vi "GUI_Magspec_BELLA_waterfall.vi"() -> ()   [LabVIEW 2013]
uses:
  shared programs/GUI_Template/GUI_master/tcp_new_data_event.ctl
  shared programs/GUI_Template/GUI_master/tcp new data cluster.ctl
  General/Device GUIs/GUI_Cameras/color tables/image color table presets.ctl
  shared programs/MySQL/Preset Query Enum.ctl
  <vilib>/Analysis/2dsp.llb/Decimate (single shot, DBL).vi
  <vilib>/Utility/tcp.llb/UDP Multicast Read-Only Open.vi
  <vilib>/vision/NI_Vision_Development_Module.lvlib
  <vilib>/Analysis/NI_AALPro.lvlib
panel:
  in  "Color table":T1=enum."BYR enhance low"
  out "Momentum 3":dbl=8.582505 caption="Momentum (GeV/c)" min=0.0 max=0.0 format="%#.1f"
  out "Momentum 4":dbl=7.19823 caption="Momentum (GeV/c)" min=0.0 max=0.0 format="%#.1f"
  out "Momentum 5":dbl=5.675527499999999 caption="Momentum (GeV/c)" min=0.0 max=0.0 format="%#.1f"
  out "Momentum 6":dbl=4.36046625 caption="Momentum (GeV/c)" min=0.0 max=0.0 format="%#.1f"
  out "C":T2(plugin-control) caption="C cam"
  out "D":T2(plugin-control) caption="D Cam"
  out "E":T2(plugin-control) caption="E Cam"
  out "Momentum 7":dbl=4.014397499999999 caption="Momentum (GeV/c)" min=0.0 max=0.0 format="%#.1f"
  out "Momentum 8":dbl=2.97619125 caption="Momentum (GeV/c)" min=0.0 max=0.0 format="%#.1f"
  out "Momentum 9":dbl=2.0210415 caption="Momentum (GeV/c)" min=0.0 max=0.0 format="%#.1f"
  out "Momentum 10":dbl=1.218162 caption="Momentum (GeV/c)" min=0.0 max=0.0 format="%#.1f"
  out "Momentum 11":dbl=0.67829475 caption="Momentum (GeV/c)" min=0.0 max=0.0 format="%#.1f"
  out "Momentum 12":dbl=0.276855 caption="Momentum (GeV/c)" min=0.0 max=0.0 format="%#.1f"
  out "Momentum 13":dbl=0.06921375 caption="Momentum (GeV/c)" min=0.0 max=0.0 format="%#.1f"
  out "Momentum 14":dbl=0.0055371 caption="Momentum (GeV/c)" min=0.0 max=0.0 format="%#.1f"
  out "F":T2(plugin-control) caption="F Cam"
  out "G":T2(plugin-control) caption="G Cam"
  out "H":T2(plugin-control) caption="H Cam"
  out "I":T2(plugin-control) caption="I Cam"
  out "J":T2(plugin-control) caption="J Cam"
  out "K":T2(plugin-control) caption="K Cam"
  out "L":T2(plugin-control) caption="L Cam"
  out "Momentum 2":dbl=9.5514975 caption="Momentum (GeV/c)" min=0.0 max=0.0 format="%#.1f"
  out "B":T2(plugin-control) caption="B Cam"
  out "Momentum 1":dbl=26.301225 caption="Momentum (GeV/c)" min=0.0 max=0.0 format="%#.1f"
  out "EBeam":T2(plugin-control) caption="Beam Profile"
  out "A":T2(plugin-control) caption="A Cam"
  in  "Max P [MeV/c]":dbl=6000.0
  out "ROI interpolated":cluster{"yi":dbl[], dbl[]}(graph)
  out "rough calcs out":T3={"peak charge (a.u.)"=nan, "momentum at peak (MeV/c)"=nan, "FWHM (MeV/c)"=nan, "Background"=nan, "sum"=0.0}
  in  "proper stitch":bool=TRUE
  out "Intensity Graph 6":dbl[][](graph)
  in  "Field::14":dbl=2.76855 caption="B Field (mT)" min=0.0 max=0.0 format="%_4f"
  out "Boolean":bool
  in  "options":T4={"B field [mT]"=400.0, "Max P [MeV/c]"=400.0, "filter rank"=1}
  out "ShotNumber":i32
  out "data":string[][](array[string])
  in  "rank for LPF":i32=2
  out "Waveform Graph":dbl[](graph)
  in  "HorizontalLineout::12":dbl[](array[numeric]) caption="HorizontalLineout MagSpecA"
  in  "HorizontalLineout::11":dbl[](array[numeric]) caption="HorizontalLineout MagSpecA"
  in  "HorizontalLineout::10":dbl[](array[numeric]) caption="HorizontalLineout MagSpecA"
  in  "HorizontalLineout::9":dbl[](array[numeric]) caption="HorizontalLineout MagSpecA"
  in  "HorizontalLineout::8":dbl[](array[numeric]) caption="HorizontalLineout MagSpecA"
  in  "HorizontalLineout::7":dbl[](array[numeric]) caption="HorizontalLineout MagSpecA"
  in  "HorizontalLineout::6":dbl[](array[numeric]) caption="HorizontalLineout MagSpecA"
  in  "HorizontalLineout::5":dbl[](array[numeric]) caption="HorizontalLineout MagSpecA"
  in  "HorizontalLineout::4":dbl[](array[numeric]) caption="HorizontalLineout MagSpecA"
  in  "HorizontalLineout::3":dbl[](array[numeric]) caption="HorizontalLineout MagSpecA"
  in  "HorizontalLineout::2":dbl[](array[numeric]) caption="HorizontalLineout MagSpecA"
  in  "HorizontalLineout::1":dbl[](array[numeric]) caption="HorizontalLineout MagSpecA"
  in  "GUIdevice 12":string="MagSpecL"
  in  "GUIdevice 11":string="MagSpecK"
  in  "GUIdevice 10":string="MagSpecJ"
  in  "GUIdevice 9":string="MagSpecI"
  in  "GUIdevice 8":string="MagSpecH"
  in  "GUIdevice 7":string="MagSpecG"
  in  "GUIdevice 6":string="MagSpecF"
  in  "GUIdevice 5":string="MagSpecE"
  in  "GUIdevice 4":string="MagSpecD"
  in  "GUIdevice 3":string="MagSpecC"
  in  "GUIdevice 2":string="MagSpecB"
  in  "GUIdevice 1":string="MagSpecA"
  in  "GUIdevice 14":string="BELLA_HallProbe"
  out "error IO 2":errorcluster
  out "tcp data event":T5
  in  "stop":bool
  # "AA side"
  # "B\nT\nM"
  # "T\no\np"
  # "Parking side"
  # "Beam Axis"
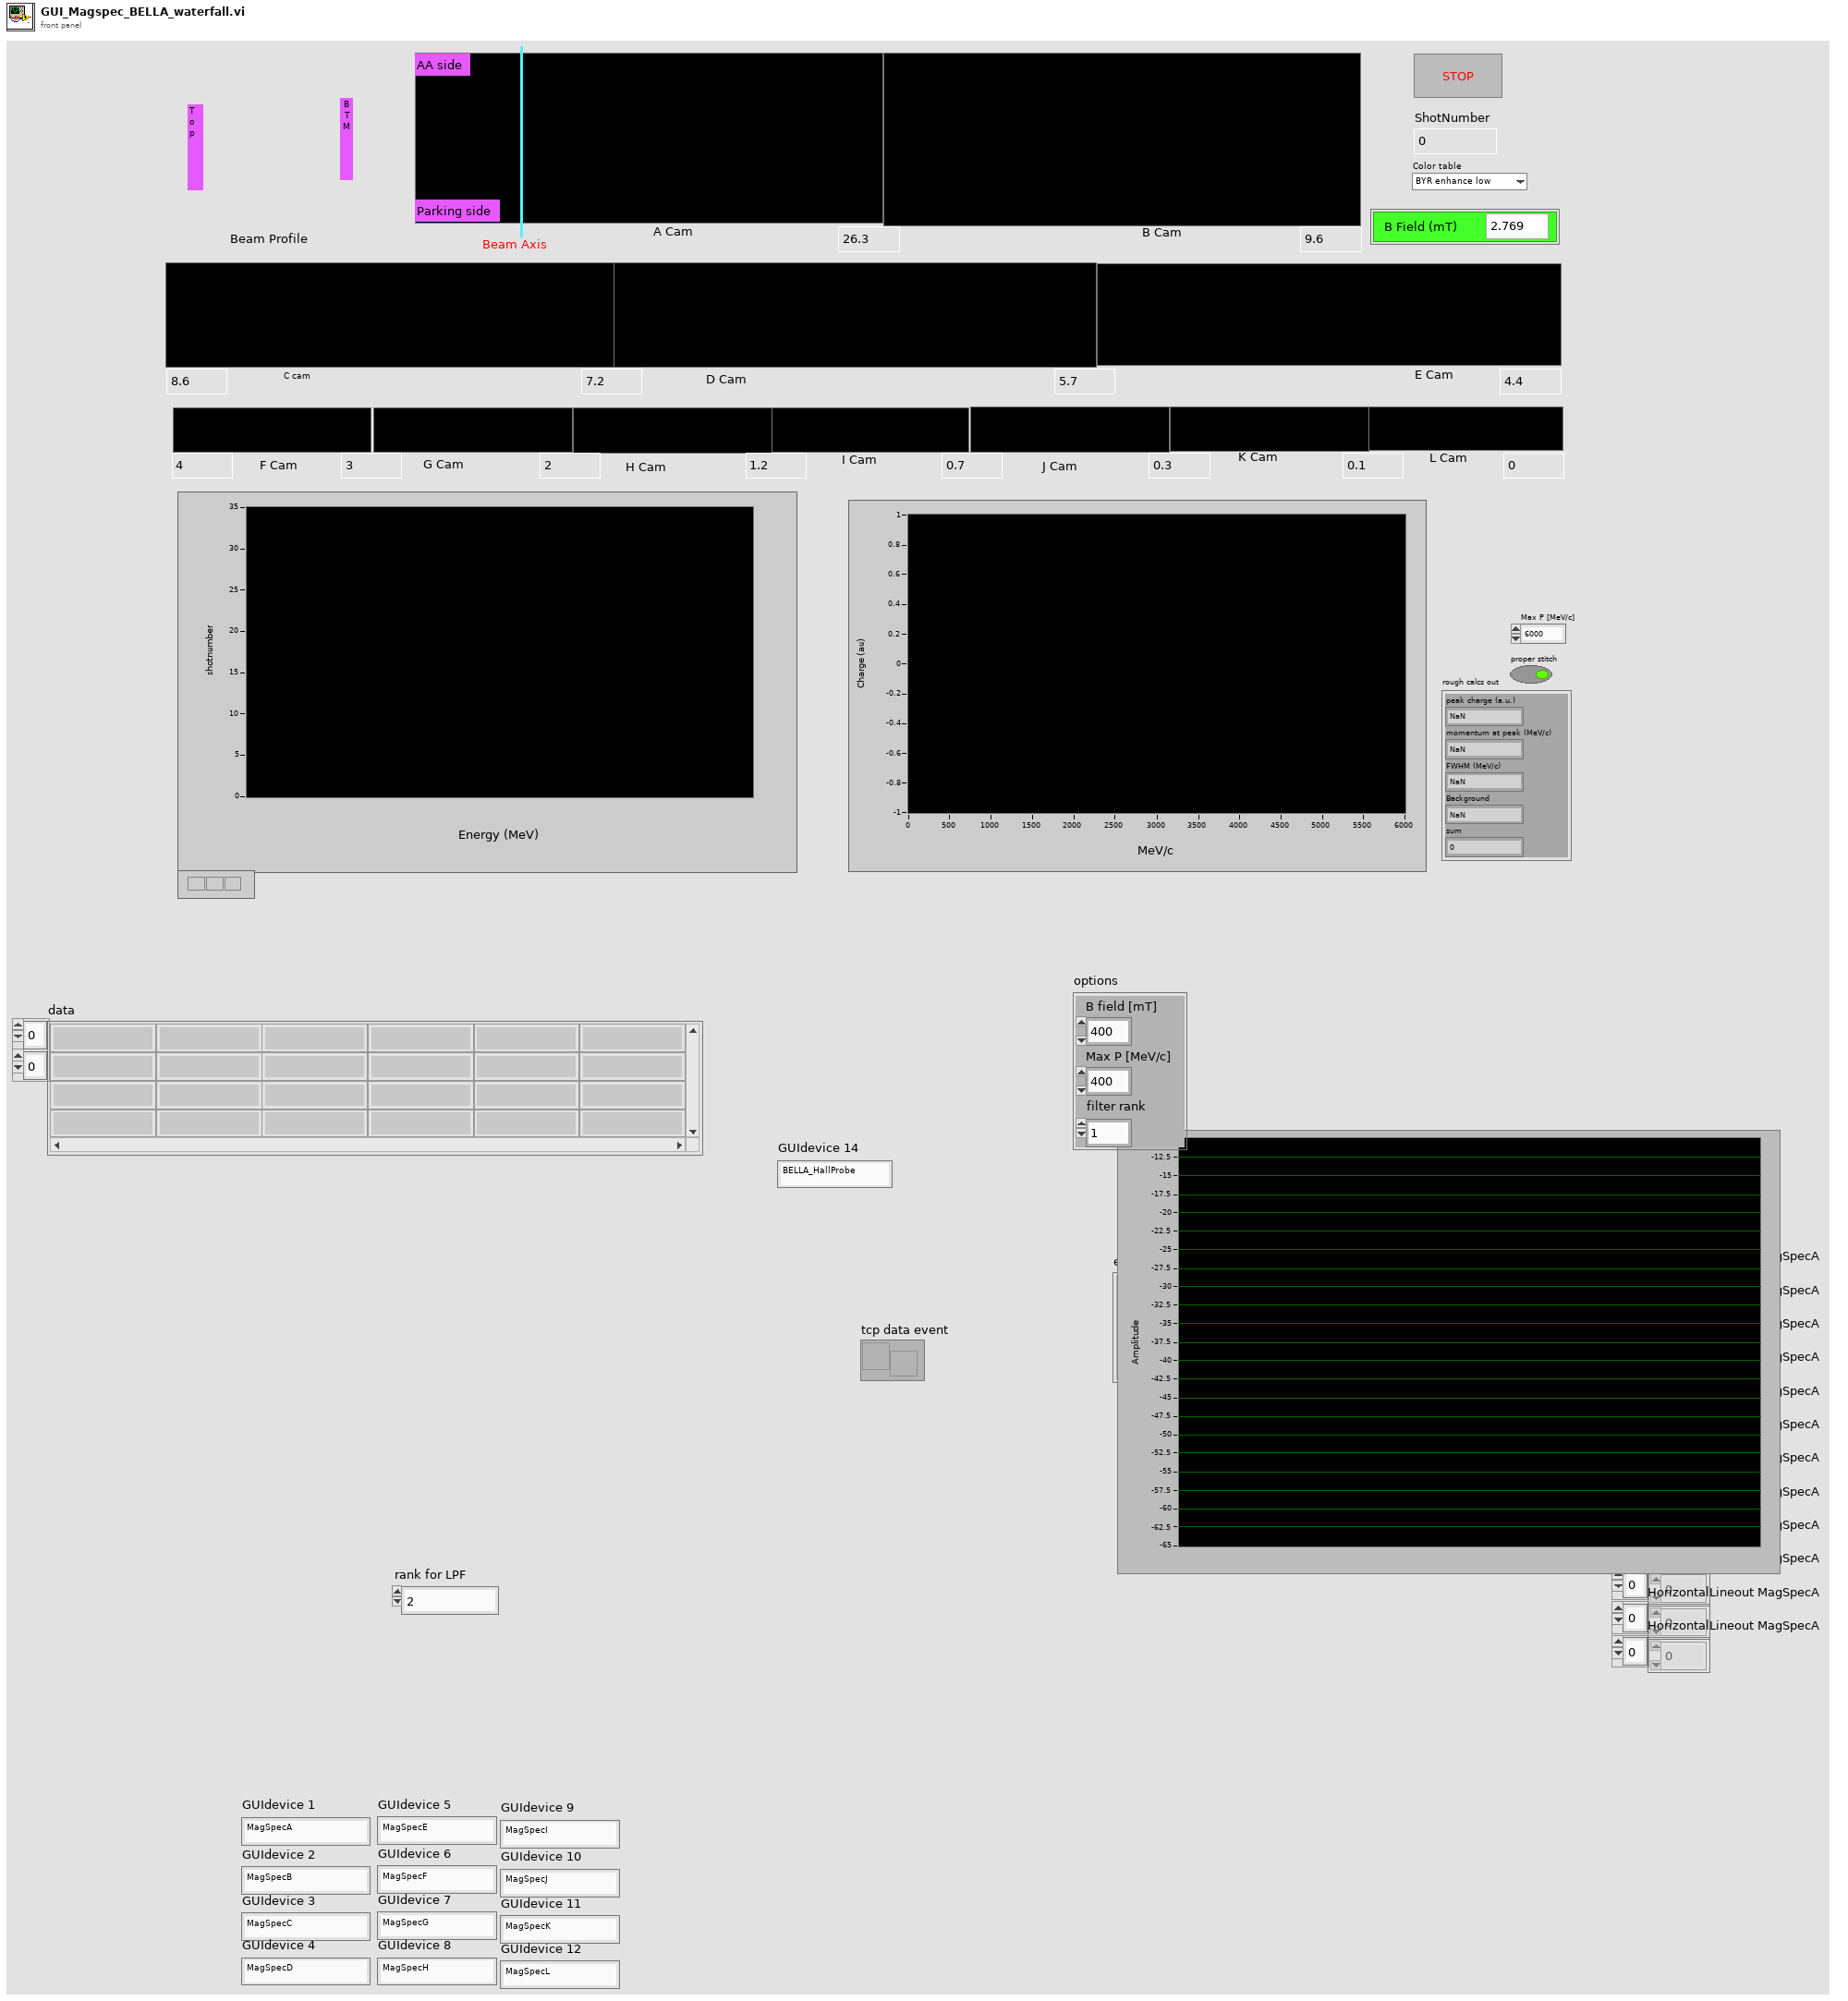
[diagram p1: front panel]
types:
  T1 = typedef "image color table presets.ctl" = enum16{"Greyscale", "Binary", "Gradient", "Rainbow", "Temperature", "enhance low", "blue yellow red", "BYR enhance low", "white blue yellow", "BWR enhance low", "make a new one"}
  T2 = typedef "IMAQ Image.ctl" = refnum<image>
  T3 = cluster{"peak charge (a.u.)":dbl, "momentum at peak (MeV/c)":dbl, "FWHM (MeV/c)":dbl, "Background":dbl, "sum":dbl}
  T4 = cluster{"B field [mT]":dbl, "Max P [MeV/c]":dbl, "filter rank":i32}
  T5 = typedef "tcp_new_data_event.ctl" = refnum<user-event>
  T6 = typedef "Image Type" = u32
  T7 = typedef "Preset Query Enum.ctl" = enum16{"Get Locations", "Get all IPs and MACs", "Get classes", "Get expt variables to set at scanstart for particular device", "Get expt devices and variables with start values", "Get expt devices and variables (with data to get)", "Get expt devices with data to get", "Get Expt devices and GUIs", "Get all devices basic properties", "Get Virtual Devices Core Info", "Get Expt names", "Get experiment basic properties", "Get experiment alarm variables", "Get MC Ports", "Get device network comm port", "Get devicetype lvclass path", "Get basic device properties", "Get Init Order", "Get all setable variables of a device", "Get device variable aliases", "Get force values of all settable variables", "Get all variables of a devicetype", "Get all variables of a device", "Get plotter details", "Get Saved Scans", "Get Scan Info", "GetGeneralGUIs", "Get expt for plotter", "Get plotter IDs from expt", "Get all devices", "Get all Virtual Devices", "Get variable and device info for Virtual Device", "GetItemLocatorIP", "Get IPs for GUIs", "Get DeviceType from Device", "GetLocalPortRange", "GetDevicePresetVariables", "Get Device Configuration", "GetAllPresetNames", "GetAllConfigurationNames", "GetPresetDeviceNames"}
  T8 = typedef "tcp new data cluster.ctl" = cluster{"EventEnum":enum16{"new data", "connection status update"}, "Device name":string}
  T9 = enum32{"invalid app kind", "Development System", "Run Time System", "Student Edition", "Embedded LabVIEW", "Evaluation", "Custom"}
  T10 = enum32{"Invalid", "Standard", "Closed", "Hidden", "Minimized", "Maximized"}
  T11 = cluster{"Core":cluster{"Current VI Reference":refnum<vi>, "Close Panel on Exit?":bool}}
  T12 = cluster{"Current VI Reference":refnum<vi>, "Close Panel on Exit?":bool}
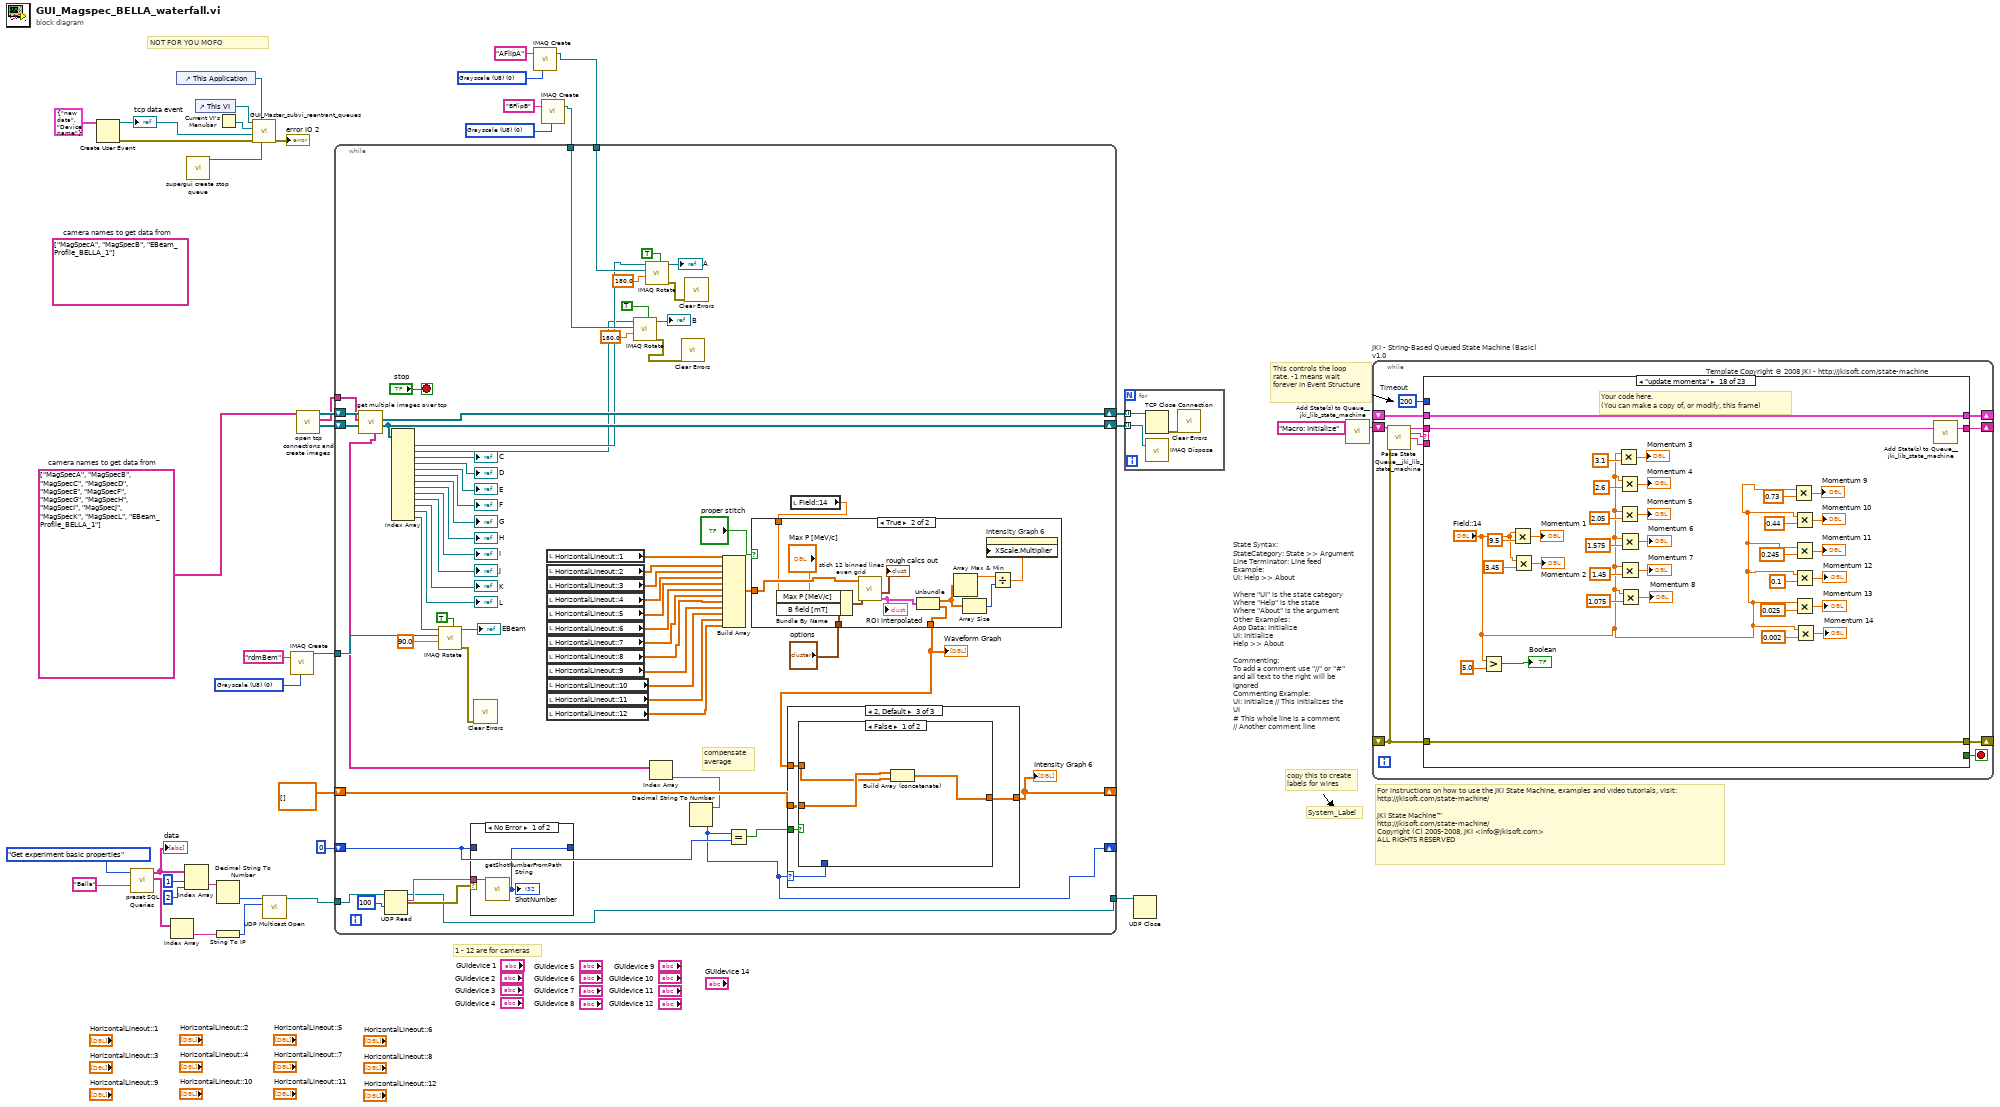
[diagram p0: block diagram]
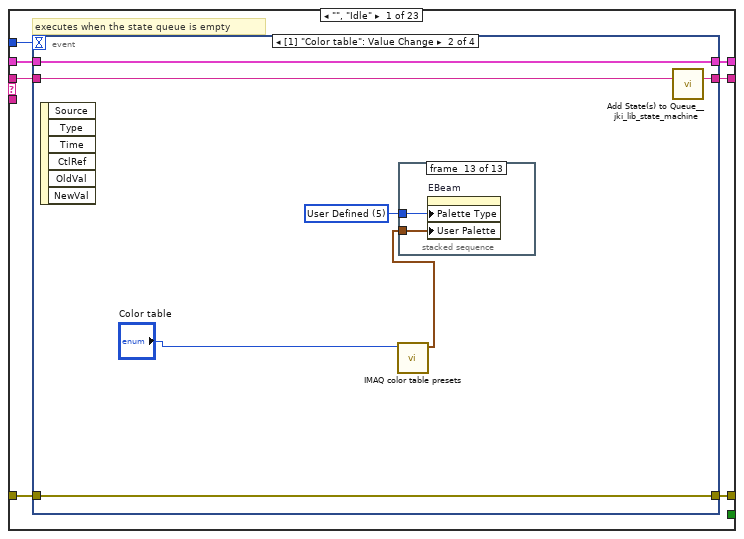
[diagram p2: hidden frame]
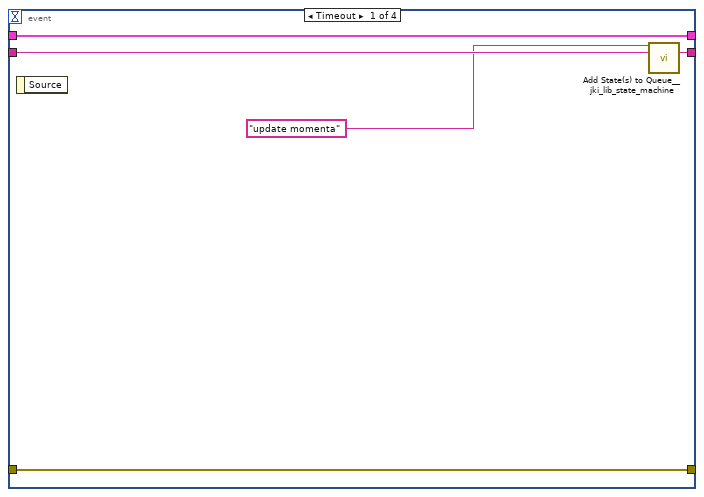
[diagram p3: hidden frame]
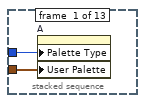
[diagram p4: hidden frame]
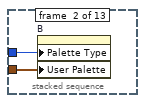
[diagram p5: hidden frame]
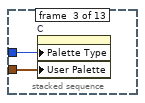
[diagram p6: hidden frame]
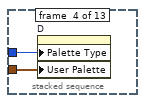
[diagram p7: hidden frame]
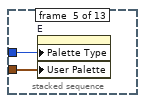
[diagram p8: hidden frame]
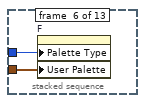
[diagram p9: hidden frame]
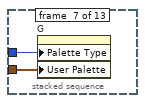
[diagram p10: hidden frame]
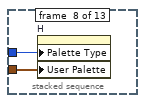
[diagram p11: hidden frame]
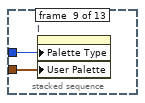
[diagram p12: hidden frame]
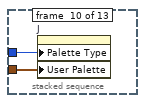
[diagram p13: hidden frame]
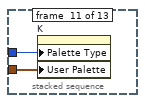
[diagram p14: hidden frame]
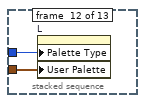
[diagram p15: hidden frame]
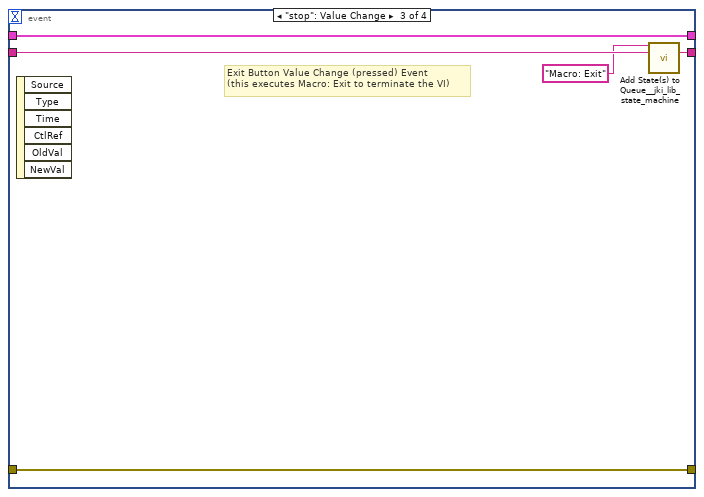
[diagram p16: hidden frame]
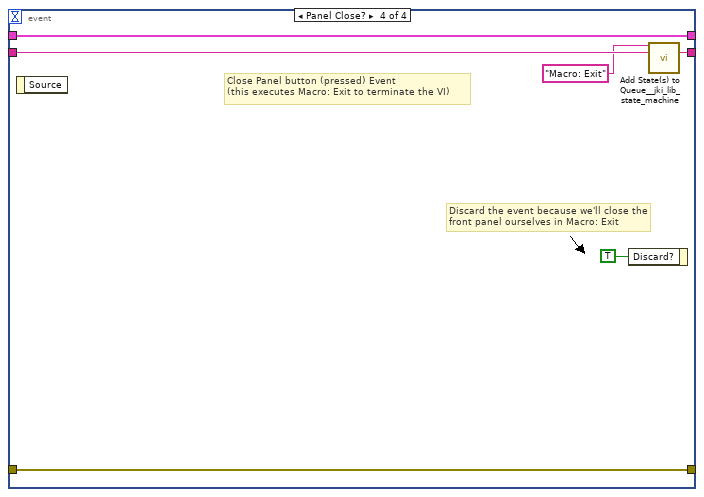
[diagram p17: hidden frame]
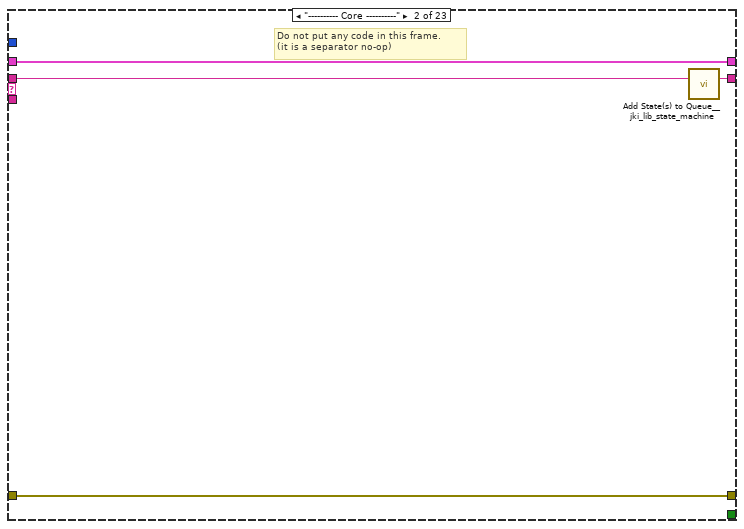
[diagram p18: hidden frame]
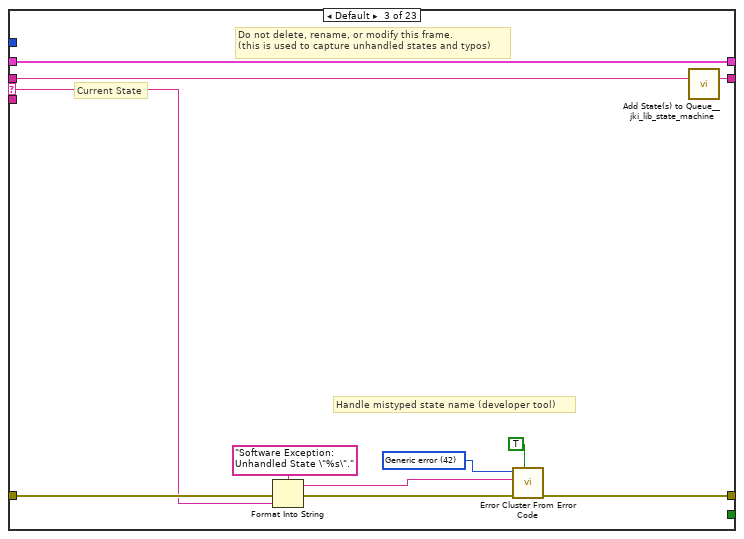
[diagram p19: hidden frame]
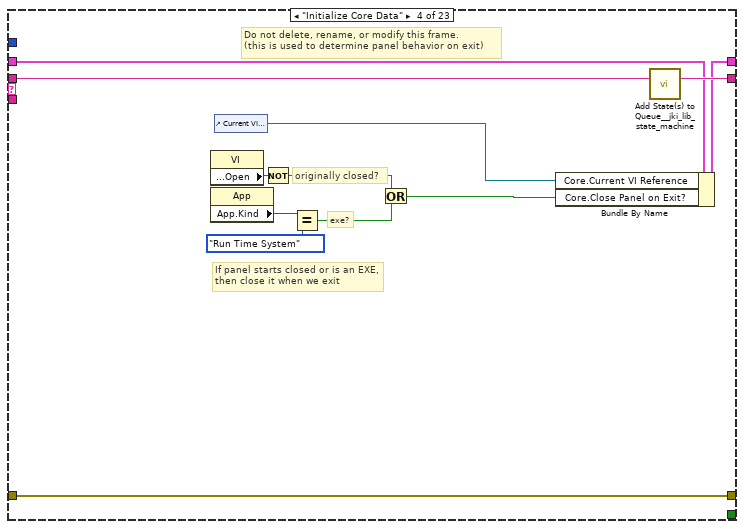
[diagram p20: hidden frame]
diagram:
  w4 = string[] ["MagSpecA", "MagSpecB", "MagSpecC", "MagSpecD", "MagSpecE", "MagSpecF", "MagSpecG", "MagSpecH", "MagSpecI", "MagSpecJ", "MagSpecK", "MagSpecL", "EBeam_Profile_BELLA_1"]  # camera names to get data from
  w8 = T6 0 items=["Grayscale (U8)", "Grayscale (I16)", "Grayscale (SGL)", "Complex (CSG)", "RGB (U32)", "HSL (U32)", "RGB (U64)", "Grayscale (U16)"] ("Image Type")
  w12 = T6 0 items=["Grayscale (U8)", "Grayscale (I16)", "Grayscale (SGL)", "Complex (CSG)", "RGB (U32)", "HSL (U32)", "RGB (U64)", "Grayscale (U16)"] ("Image Type")
  w14 = T6 0 items=["Grayscale (U8)", "Grayscale (I16)", "Grayscale (SGL)", "Complex (CSG)", "RGB (U32)", "HSL (U32)", "RGB (U64)", "Grayscale (U16)"] ("Image Type")
  (unwired) string[] ["MagSpecA", "MagSpecB", "EBeam_Profile_BELLA_1"]  # camera names to get data from
  # "For instructions on how to use the JKI State Machine, examples and video tutorials, visit:\nhttp://jkisoft.com/state-machine/\n\nJKI State Machine™\nhttp://jkisoft.com/state-machine/\nCopyright (C) 2005-2008, JKI <info@jkisoft.com>\nALL RIGHTS RESERVED"
  # "State Syntax:\nStateCategory: State >> Argument\nLine Terminator: Line feed\nExample:\nUI: Help >> About\n\nWhere \"UI\" is the state category\nWhere \"Help\" is the state\nWhere \"About\" is the argument\nOther Examples:\nApp Data: Initialize\nUI: Initialize\nHelp >> About\n\nCommenting:\nTo add a comment use \"//\" or \"#\" and all text to the right will be ignored\nCommenting Example:\nUI: Initialize // This initializes the UI\n# This whole line is a comment\n// Another comment line"
  # "copy this to create labels for wires"
  # "This controls the loop rate. -1 means wait forever in Event Structure"
  # "System_Label"
  # "1 - 12 are for cameras"
  # "NOT FOR YOU MOFO"
  n1 = Create User Event(user event datatype=T8 {"EventEnum"=enum."new data", "Device name"="Device name"} ("New Event")) -> (user event=w29:refnum<user-event>, error out=w30:errorcluster)  [unwired: 1 in]
  "tcp data event" <- w29
  n2 = call "preset SQL Queries.vi"("Expt name / MCIP/ Variable/Preset Name"="Bella", "Preset Query"=Preset_Query_Enum."Get experiment basic properties") -> ("1st column 1st data"=w20:string[], "data"=w21:string[][])  [unwired: 7 in, 1 out]
  "data" <- w21
  n3 = Index Array(array=w20) -> (element=w19:string)  [unwired: 1 in]
  n4 = control-ref of="This Application"() -> (w28:refnum<vi>)
  n5 = Index Array(array=w21, index (row)=1, index (col)=2 ("disabled index (col)")) -> (element=w22:string)
  n6 = call "supergui create stop queue.vi"() -> ("STOP Queue out"=w1:refnum<queue>)  [unwired: 11 in]
  n7 = control-ref of="This VI"() -> (w33:refnum<vi>)
  n8 = Decimal String To Number(string=w22) -> (number=w18:i32)  [unwired: 2 in, 1 out]
  n9 = String To IP(1:w19) -> (0:w25:u32)
  n10 = Current VI's Menubar() -> (w32:refnum<k9>)
  n11 = call "GUI_Master_subvi_reentrant_queues.vi"("STOP Queue in"=w1, "This Application"=w28, "error in (no error)"=w30, "tcp data event"=w29, "Caller menu reference"=w32, "Caller VI ref"=w33) -> ("error out"=→"error IO 2":errorcluster)  [unwired: 5 in]
  n12 = call-poly <vilib>:"UDP Multicast Open.vi"("multicast addr"=w25, "port"=w18) -> ("connection ID"=w17:refnum<k16>)  [unwired: 7 in, 2 out]
  n13 = call "IMAQ Create"("Image Name"="rdmBem", "Image Type"=w8) -> ("New Image"=w7:T2)  [unwired: 3 in, 1 out]
  n14 = call "open tcp connections and create images.vi"("devices to get data from"=w4) -> ("images"=w36:T2[], "subscribe messages\nfor process vis"=w37:string[], "tcp connections"=w38:refnum<k5>[])  [unwired: 8 in]
  n15 = call "IMAQ Create"("Image Name"="AFlipA", "Image Type"=w14) -> ("New Image"=w13:T2)  [unwired: 3 in, 1 out]
  n16 = call "IMAQ Create"("Image Name"="BFlipB", "Image Type"=w12) -> ("New Image"=w10:T2)  [unwired: 3 in, 1 out]
  n17 = while {
    shift-right: [w100] -> w39
    shift-left: w38 -> [w101]
    tunnel: w37 -> [w99]
    shift-right: [w44] -> w35
    shift-left: w36 -> [w98]
    tunnel: w17 -> [w69]
    tunnel: [w68] -> w16
    tunnel: w13 -> [w67]
    tunnel: w10 -> [w66]
    tunnel: w7 -> [w65]
    shift-right: [w62] -> _
    shift-left: dbl[][] [] ("wavelength 2") -> [w63]
    shift-right: [w55] -> _
    shift-left: 0 ("ShotNumber") -> [w56]
    stop <- "stop" stop-if-true
    # "compensate\naverage"
    n18 = call "get multiple images over tcp.vi"("images In"=w98, "subscribeMessages"=w99, "TCP_Refs In"=w101) -> ("Images out"=w44:T2[], "TCP_Refs_out"=w100:refnum<k5>[], "shot numbers"=w58:string[])  [unwired: 4 in, 2 out]
    n19 = UDP Read(connection ID=w69, timeout ms (25000)=100) -> (data out=w71:string, error out=w70:errorcluster, 3:w68:refnum<k16>)  [unwired: 1 in, 3 out]
    n20 = Index Array(array=w44) -> (element #1=w43:T2, element #2=w42:T2, element #3=→"C":T2, element #4=→"D":T2, element #5=→"E":T2, element #6=→"F":T2, element #7=→"G":T2, element #8=→"H":T2, element #9=→"I":T2, element #10=→"J":T2, element #11=→"K":T2, element #12=→"L":T2, element #13=w41:T2)  [unwired: 13 in]
    n21 = call "IMAQ Rotate"("Maintain Size"=TRUE, "Angle (degrees)"=sgl 90.0, "Image Dst"=w65, "Image Src"=w41) -> ("error out"=w88:errorcluster, "Image Dst Out"=→"EBeam":T2)  [unwired: 6 in]
    n22 = case shown="No Error" w70 {
      selector: w70 -> [_ w140]
      tunnel: w71 -> [w138 _]
      tunnel: w56 -> [_ w139]
      tunnel: [w137 w139] -> _
      frame No Error {
        n23 = call "getShotNumberFromPathString.vi"("Path String"=w138) -> ("ShotNumber from path"=w137:i32)
        "ShotNumber" <- w137
      }
      frame Error {
        n24 = call <vilib>:"Clear Errors.vi"("error in (no error)"=w140) -> ()  [unwired: 6 in, 1 out]
      }
    }
    n25 = call <vilib>:"Clear Errors.vi"("error in (no error)"=w88) -> ()  [unwired: 6 in, 1 out]
    n26 = local read "HorizontalLineout::1"() -> (w85:dbl[])
    n27 = local read "HorizontalLineout::2"() -> (w84:dbl[])
    n28 = local read "HorizontalLineout::3"() -> (w83:dbl[])
    n29 = local read "HorizontalLineout::4"() -> (w82:dbl[])
    n30 = local read "HorizontalLineout::5"() -> (w81:dbl[])
    n31 = local read "HorizontalLineout::6"() -> (w80:dbl[])
    n32 = local read "HorizontalLineout::7"() -> (w79:dbl[])
    n33 = local read "HorizontalLineout::8"() -> (w78:dbl[])
    n34 = local read "HorizontalLineout::9"() -> (w77:dbl[])
    n35 = local read "HorizontalLineout::10"() -> (w76:dbl[])
    n36 = local read "HorizontalLineout::11"() -> (w75:dbl[])
    n37 = local read "HorizontalLineout::12"() -> (w74:dbl[])
    n38 = call "IMAQ Rotate"("Maintain Size"=TRUE, "Angle (degrees)"=sgl 180.0, "Image Dst"=w66, "Image Src"=w42) -> ("error out"=w87:errorcluster, "Image Dst Out"=→"B":T2)  [unwired: 6 in]
    n39 = call "IMAQ Rotate"("Maintain Size"=TRUE, "Angle (degrees)"=sgl 180.0, "Image Dst"=w67, "Image Src"=w43) -> ("error out"=w86:errorcluster, "Image Dst Out"=→"A":T2)  [unwired: 6 in]
    n40 = Index Array(array=w58) -> (element=w57:string)  [unwired: 1 in]
    n41 = call <vilib>:"Clear Errors.vi"("error in (no error)"=w87) -> ()  [unwired: 6 in, 1 out]
    n42 = call <vilib>:"Clear Errors.vi"("error in (no error)"=w86) -> ()  [unwired: 6 in, 1 out]
    n43 = Decimal String To Number(string=w57) -> (number=w55:i32)  [unwired: 2 in, 1 out]
    n44 = Build Array(w85, w84, w83, w82, w81, w80, w79, w78, w77, w76, w75, w74) -> (w73:dbl[][])
    n45 = Equal?(x=w55, y=w56) -> (x = y?=w59:bool)
    n46 = local read "Field::14"() -> (w40:dbl)
    n47 = case shown="True" "proper stitch" {
      tunnel: w73 -> [w111 w120]
      tunnel: [w103 w114] -> w64
      tunnel: "options" -> [_ w123]
      tunnel: w40 -> [_ w113]
      frame False {
        w105 = 8 ("decimating factor")
        n48 = Reshape Array(w111, 16608 ("dimension size")) -> (w109:dbl[])
        n49 = call-poly <vilib>:"Decimate (single shot).vi"("averaging"=TRUE, "decimating factor"=w105, "X"=w109) -> ("Decimated Array"=w106:dbl[])  [unwired: 7 in, 1 out]
        n50 = Multiply(x=w106, y=w105) -> (x*y=w107:dbl[])
        n51 = call "stich 12 binned lines online.vi"("rank"="rank for LPF", "Input"=w107) -> ("stiched signal"=w103:dbl[])
      }
      frame True {
        n52 = Bundle By Name(cluster=w123, "Max P [MeV/c]"="Max P [MeV/c]", "B field [mT]"=w113) -> (w122:T4)
        n53 = call "stich 12 binned lines even grid.vi"("options"=w122, "data in"=w120) -> ("ROI interpolated"=w116:cluster{"yi":dbl[], dbl[]}, "rough calcs out"=→"rough calcs out":T3)  [unwired: 2 in, 2 out]
        "ROI interpolated" <- w116
        n54 = Unbundle(w116) -> ("yi"=w115:dbl[], w114:dbl[])
        n55 = Array Max & Min(array=w115) -> (max value=w119:dbl)  [unwired: 3 out]
        n56 = Array Size(array=w115) -> (size(s)=w118:i32)
        n57 = Divide(x=w119, y=w118) -> (x/y=w117:dbl)
        n58 = property on="Intensity Graph 6" class="IntGraph (strict)"("XScale.Multiplier"=w117) -> ()  [unwired: 2 in, 2 out]
      }
    }
    "Waveform Graph" <- w64
    n59 = case shown="2, Default" w55 {
      selector: w55 -> [_ _ w128]
      tunnel: w63 -> [_ w127 w132]
      tunnel: w64 -> [w125 _ w131]
      tunnel: [w124 w127 w130] -> w62
      tunnel: w59 -> [_ _ w129]
      frame 1 {
        n60 = Build Array (concatenate)(dbl[][] [] ("wavelength 2"), w125) -> (w124:dbl[][])
      }
      frame 0 {
      }
      frame 2, Default {
        n61 = case shown="False" w129 {
          tunnel: w132 -> [w135 w136]
          tunnel: w131 -> [w134 _]
          tunnel: [w133 w136] -> w130
          tunnel: w128 -> [_ _]
          frame False {
            n62 = Build Array (concatenate)(w135, w134) -> (w133:dbl[][])
          }
          frame True {
          }
        }
      }
    }
    "Intensity Graph 6" <- w62
  }
  n63 = for {
    tunnel: w39 -> [w143] mode=indexing
    tunnel: w35 -> [w142] mode=indexing
    n64 = TCP Close Connection(connection ID=w143) -> (error out=w141:errorcluster)  [unwired: 2 in, 1 out]
    n65 = call "IMAQ Dispose"("Image"=w142) -> ()  [unwired: 5 in, 1 out]
    n66 = call <vilib>:"Clear Errors.vi"("error in (no error)"=w141) -> ()  [unwired: 6 in, 1 out]
  }
  n67 = UDP Close(connection ID=w16) -> ()  [unwired: 1 in, 2 out]
  n68 = call <vilib>:"Add State(s) to Queue__jki_lib_state_machine.vi"("State(s) in (\"\")"="Macro: Initialize") -> ("States Out"=w3:string)  [unwired: 14 in]
  n69 = while "JKI - String-Based Queued State Machine (Basic) v1.0" {
    shift-right: [w147] -> _
    shift-left: _ -> [w146]
    shift-right: [w150] -> _
    shift-left: _ -> [w144]
    shift-right: [w149] -> _
    shift-left: w3 -> [w151]
    stop <- w148 stop-if-true
    w145 = 200  # Timeout
    # "Template Copyright © 2008 JKI - http://jkisoft.com/state-machine"
    n70 = call <vilib>:"Parse State Queue__jki_lib_state_machine.vi"("State Queue"=w151, "Error In (no error)"=w144) -> ("Remaining States"=w153:string, "Current State"=w154:string, "Arguments"=w152:string)  [unwired: 11 in]
    n71 = case shown="\"update momenta\"" w154 {
      selector: w154 -> [_ _ w215 _ _ _ _ _ _ _ _ _ _ _ _ _ _ _ _ _ _ _ _]
      tunnel: w153 -> [w161 w214 w219 w237 w243 w248 w252 w258 w264 w268 w272 w278 w289 w315 w320 w330 w334 w369 w373 w377 w381 w385 w389]
      tunnel: w152 -> [_ _ _ _ _ _ _ _ _ _ _ w273 w283 _ _ _ _ _ _ _ _ _ _]
      tunnel: w146 -> [w159 w211 w217 w228 w240 w246 w249 _ w259 w265 w270 w276 w285 w312 w317 w327 w331 w366 w370 w374 w378 w382 w386]
      tunnel: [w158 w212 w221 w234 errorcluster {"status"=FALSE, "code"=0, "source"=""} ("error out") w245 w250 w255 w260 w266 w269 w274 w286 w313 w318 w328 w332 w367 w371 w375 w379 w383 w387] -> w150
      tunnel: w144 -> [w157 w212 w220 w234 w239 w245 w250 w255 w261 w266 w269 w275 w287 w313 w318 w328 w332 w367 w371 w375 w379 w383 w387]
      tunnel: [w160 w213 w218 w236 w242 w247 w251 w257 w263 w267 w271 w277 w288 w314 w319 w329 w333 w368 w372 w376 w380 w384 w388] -> w149
      tunnel: [_ _ _ _ _ TRUE _ _ _ _ _ _ _ _ _ _ _ _ _ _ _ _ _] -> w148
      tunnel: [w156 w211 w217 w235 w240 w246 w249 w256 w259 w265 w270 w276 w285 w312 w317 w327 w331 w366 w370 w374 w378 w382 w386] -> w147
      tunnel: w145 -> [w155 _ _ _ _ _ _ _ _ _ _ _ _ _ _ _ _ _ _ _ _ _ _]
      frame "", "Idle" {
        # "executes when the state queue is empty"
        n72 = event shown="[1] \"Color table\": Value Change" {
          selector: _ -> [_ _ _ _]
          dyn-events: _ -> [_ _ _ _]
          timeout: w155 -> [_ _ _ _]
          tunnel: w161 -> [w166 w173 w204 w210]
          tunnel: [w165 w172 w203 w209] -> w160
          tunnel: w159 -> [w163 w170 w201 w207]
          tunnel: [w164 w171 w202 w208] -> w158
          tunnel: w157 -> [w164 w171 w202 w208]
          tunnel: [w163 w170 w201 w207] -> w156
          event Timeout {
            n73 = event-data() -> ()  [unwired: 1 in, 1 out]
            n74 = call <vilib>:"Add State(s) to Queue__jki_lib_state_machine.vi"("State(s) in Front (\"\")"="update momenta" ("State(s) in Front (\"\")"), "State(s) in (\"\")"=w166) -> ("States Out"=w165:string)  [unwired: 13 in]
          }
          event Value Change {
            w169 = u32 5 items=["Grayscale", "Binary", "Gradient", "Rainbow", "Temperature", "User Defined"] ("Palette:Palette Type")
            n75 = event-data() -> ()  [unwired: 1 in, 6 out]
            n76 = call "IMAQ color table presets.vi"("Color table"="Color table") -> ("Array"=w167:cluster{"R":u8, "G":u8, "B":u8}[])  [unwired: 9 in, 1 out]
            n77 = stacked-sequence {
              tunnel: w169 -> [w175 w177 w179 w181 w183 w185 w187 w189 w191 w193 w195 w197 w199]
              tunnel: w167 -> [w174 w176 w178 w180 w182 w184 w186 w188 w190 w192 w194 w196 w198]
              frame #0 {
                n78 = property on="A" class="ImageControl"("Palette Type"=w175, "User Palette"=w174) -> ()  [unwired: 2 in, 2 out]
              }
              frame #1 {
                n79 = property on="B" class="ImageControl"("Palette Type"=w177, "User Palette"=w176) -> ()  [unwired: 2 in, 2 out]
              }
              frame #2 {
                n80 = property on="C" class="ImageControl"("Palette Type"=w179, "User Palette"=w178) -> ()  [unwired: 2 in, 2 out]
              }
              frame #3 {
                n81 = property on="D" class="ImageControl"("Palette Type"=w181, "User Palette"=w180) -> ()  [unwired: 2 in, 2 out]
              }
              frame #4 {
                n82 = property on="E" class="ImageControl"("Palette Type"=w183, "User Palette"=w182) -> ()  [unwired: 2 in, 2 out]
              }
              frame #5 {
                n83 = property on="F" class="ImageControl"("Palette Type"=w185, "User Palette"=w184) -> ()  [unwired: 2 in, 2 out]
              }
              frame #6 {
                n84 = property on="G" class="ImageControl"("Palette Type"=w187, "User Palette"=w186) -> ()  [unwired: 2 in, 2 out]
              }
              frame #7 {
                n85 = property on="H" class="ImageControl"("Palette Type"=w189, "User Palette"=w188) -> ()  [unwired: 2 in, 2 out]
              }
              frame #8 {
                n86 = property on="I" class="ImageControl"("Palette Type"=w191, "User Palette"=w190) -> ()  [unwired: 2 in, 2 out]
              }
              frame #9 {
                n87 = property on="J" class="ImageControl"("Palette Type"=w193, "User Palette"=w192) -> ()  [unwired: 2 in, 2 out]
              }
              frame #10 {
                n88 = property on="K" class="ImageControl"("Palette Type"=w195, "User Palette"=w194) -> ()  [unwired: 2 in, 2 out]
              }
              frame #11 {
                n89 = property on="L" class="ImageControl"("Palette Type"=w197, "User Palette"=w196) -> ()  [unwired: 2 in, 2 out]
              }
              frame #12 {
                n90 = property on="EBeam" class="ImageControl"("Palette Type"=w199, "User Palette"=w198) -> ()  [unwired: 2 in, 2 out]
              }
            }
            n91 = call <vilib>:"Add State(s) to Queue__jki_lib_state_machine.vi"("State(s) in (\"\")"=w173) -> ("States Out"=w172:string)  [unwired: 14 in]
          }
          event "stop": Value Change {
            # "Exit Button Value Change (pressed) Event\n(this executes Macro: Exit to terminate the VI)"
            n92 = event-data() -> ()  [unwired: 1 in, 6 out]
            n93 = call <vilib>:"Add State(s) to Queue__jki_lib_state_machine.vi"("State(s) in Front (\"\")"="Macro: Exit", "State(s) in (\"\")"=w204) -> ("States Out"=w203:string)  [unwired: 13 in]
          }
          event Panel Close? {
            # "Discard the event because we'll close the front panel ourselves in Macro: Exit"
            # "Close Panel button (pressed) Event\n(this executes Macro: Exit to terminate the VI)"
            n94 = event-data() -> ()  [unwired: 1 in, 1 out]
            n95 = event-data("Discard?"=TRUE) -> ()  [unwired: 1 in, 1 out]
            n96 = call <vilib>:"Add State(s) to Queue__jki_lib_state_machine.vi"("State(s) in Front (\"\")"="Macro: Exit", "State(s) in (\"\")"=w210) -> ("States Out"=w209:string)  [unwired: 13 in]
          }
        }
      }
      frame "---------- Core ----------" {
        # "Do not put any code in this frame.\n(it is a separator no-op)"
        n97 = call <vilib>:"Add State(s) to Queue__jki_lib_state_machine.vi"("State(s) in (\"\")"=w214) -> ("States Out"=w213:string)  [unwired: 14 in]
      }
      frame Default {
        w224 = 42 items=["No error", "Argument error", "Memory is full", "Out of zone", "End of file", "File already open", "Generic file I/O error", "File not found", "File permission error", "Disk is full", "Duplicate path", "Too many files open", "System feature not enabled", "Resource file not found", "Cannot add resource", "Resource not found", "Image not found", "Image memory error", "Pen does not exist", "Config type invalid", "Config token not found", "Config parse error", "Config memory error", "Bad external code format", "Bad external code offset", "External code not present", "Null window", "Destroy window error", "Null menu", "Print aborted", "Bad print record", "Print driver error", "Windows error during printing", "Memory error during printing", "Print dialog error", "Generic print error", "Invalid device refnum", "Device not found", "Device parameter error", "Device unit error", "Cannot open device", "Device call aborted", "Generic error", "Cancelled by user", "Object ID too low", "Object ID too high", "Object not in heap", "Unknown heap", "Unknown object (invalid DefProc)", "Unknown object (DefProc not in table)", "Message out of range", "Invalid (null) method", "Unknown message", "Manager call not supported", "Bad address", "Network operation in progress", "Network operation timed out", "Connection is busy", "Network attribute not supported", "Network error", "Address in use", "System out of memory", "Connection aborted", "Connection refused", "Not connected", "Already connected", "Connection closed", "Initialization error (interapplication manager)", "Bad occurrence", "Wait on unbound occurrence handler", "Occurrence queue overflow", "Datalog type conflict", "Unused", "Unrecognized type (interapplication manager)", "Memory corrupt", "Failed to make temporary DLL", "Old CIN version", "Drag socket not found", "Failed to load drop-object", "Failed to register OLE object", "Failed to release OLE object", "Format specifier type mismatch", "Unknown format specifier", "Too few format specifiers", "Too many format specifiers", "Scan failed", "Newer CIN version", "Error converting to variant", "Runtime menu error", "Password tampered", "Variant attribute not found", "Incompatible variant data type", "Event data is not available", "Event Store is not present", "Occurrence is not found", "Event Queue is not created", "Event info is not available", "Refnum passed is NULL", "Error retrieving Class GUID", "Error retrieving CoClass GUID", "Error retrieving TypeLib GUID.", "Bad built application magic bytes.", "Specific driver is different from the specific driver associated with the Logical Name.", "There is no session opened to the class driver.", "Max Error", "MAX - Error with config objects", "MAX - Error loading configuration", "MAX - Group not supported"]
        # "Current State"
        # "Do not delete, rename, or modify this frame.\n(this is used to capture unhandled states and typos)"
        # "Handle mistyped state name (developer tool)"
        n98 = Format Into String(format string="Software Exception: Unhandled State \"%s\"." ("message"), error in=w220, w215) -> (resulting string=w223:string, error out=w222:errorcluster)  [unwired: 1 in]
        n99 = call <vilib>:"Error Cluster From Error Code.vi"("show call chain? (False)"=TRUE, "error in (no error)"=w222, "error message (\"\")"=w223, "error code (0)"=w224) -> ("error out"=w221:errorcluster)  [unwired: 5 in]
        n100 = call <vilib>:"Add State(s) to Queue__jki_lib_state_machine.vi"("State(s) in (\"\")"=w219) -> ("States Out"=w218:string)  [unwired: 14 in]
      }
      frame "Initialize Core Data" {
        # "Do not delete, rename, or modify this frame.\n(this is used to determine panel behavior on exit)"
        # "originally closed?"
        # "exe?"
        # "If panel starts closed or is an EXE, then close it when we exit"
        n101 = property class="VI"() -> ("Front Panel.Open"=w233:bool)  [unwired: 2 in, 2 out]
        n102 = property class="App"() -> ("App.Kind"=w232:T9)  [unwired: 2 in, 2 out]
        n103 = control-ref of="Current VI Reference"() -> (w226:refnum<vi>)
        n104 = Not(x=w233) -> (.not. x?=w230:bool)
        n105 = Equal?(x=w232, y=T9."Run Time System" ("Application:Kind")) -> (x = y?=w229:bool)
        n106 = Or(x=w230, y=w229) -> (x .or. y?=w227:bool)
        n107 = Bundle By Name(cluster=w228, "Core.Current VI Reference"=w226, "Core.Close Panel on Exit?"=w227) -> (w235:T11)
        n108 = call <vilib>:"Add State(s) to Queue__jki_lib_state_machine.vi"("State(s) in (\"\")"=w237) -> ("States Out"=w236:string)  [unwired: 14 in]
      }
      frame "Error Handler" {
        # "Unhandled Error -- Display it"
        # "Handle any errors here.\nYou can also output any states to clean-up after errors occur"
        # "Clear error"
        n109 = call <vilib>:"General Error Handler.vi"("error in (no error)"=w239) -> ()  [unwired: 10 in, 5 out]
        n110 = call <vilib>:"Add State(s) to Queue__jki_lib_state_machine.vi"("State(s) in Front (\"\")"="/* Post Error States", "State(s) in (\"\")"=w243) -> ("States Out"=w242:string)  [unwired: 13 in]
      }
      frame "Exit" {
        # "Do not put any code in this frame.\n(No errors that occur here will be handled.)"
        n111 = call <vilib>:"Add State(s) to Queue__jki_lib_state_machine.vi"("State(s) in (\"\")"=w248) -> ("States Out"=w247:string)  [unwired: 14 in]
      }
      frame "---------- Data ----------" {
        # "Do not put any code in this frame.\n(It is a separator no-op. You can make a copy of this frame to create a new Data frame)"
        n112 = call <vilib>:"Add State(s) to Queue__jki_lib_state_machine.vi"("State(s) in (\"\")"=w252) -> ("States Out"=w251:string)  [unwired: 14 in]
      }
      frame "Data: Initialize" {
        w254 = T12 {"Current VI Reference"=refnum, "Close Panel on Exit?"=FALSE}  # Core
        # "Initialize the shift-register data, here.\n(data names are defined by what you wire into the bundle function)"
        n113 = property on="Color table" class="Enum (strict)"("Val(Sgnl)"=image_color_table_presets."enhance low" ("Value (Signaling)")) -> ()  [unwired: 2 in, 2 out]
        n114 = Bundle("Core"=w254) -> (w256:T11)  [unwired: 1 in]
        n115 = call <vilib>:"Add State(s) to Queue__jki_lib_state_machine.vi"("State(s) in (\"\")"=w258) -> ("States Out"=w257:string)  [unwired: 14 in]
      }
      frame "Data: Cleanup" {
        # "Cleanup any data and references, here.\n(this is called automatically, by the Macro: Exit)"
        n116 = Unbundle By Name(w259) -> ("Core.Current VI Reference"=w262:refnum<vi>)
        n117 = Close Reference(reference=w262, error in (no error)=w261) -> (error out=w260:errorcluster)
        n118 = call <vilib>:"Add State(s) to Queue__jki_lib_state_machine.vi"("State(s) in (\"\")"=w264) -> ("States Out"=w263:string)  [unwired: 14 in]
      }
      frame "---------- UI ----------" {
        # "Do not put any code in this frame.\n(It is a separator no-op. You can make a copy of this frame to create a new UI frame)"
        n119 = call <vilib>:"Add State(s) to Queue__jki_lib_state_machine.vi"("State(s) in (\"\")"=w268) -> ("States Out"=w267:string)  [unwired: 14 in]
      }
      frame "UI: Initialize" {
        # "Initialize the User Interface, here.\n(this is called automatically, by the Macro: Init)"
        n120 = call <vilib>:"Add State(s) to Queue__jki_lib_state_machine.vi"("State(s) in (\"\")"=w272) -> ("States Out"=w271:string)  [unwired: 14 in]
      }
      frame "UI: Cursor Set" {
        # "Argument"
        # "Set and Unset Cursor Busy.\n(Usage: \"UI: Cursor Set >> Busy|Idle\")"
        n121 = case shown="\"Idle\", Default" w273 {
          tunnel: w275 -> [w280 w282]
          tunnel: [w279 w281] -> w274
          frame "Idle", Default {
            n122 = call <vilib>:"Unset Busy.vi"("error in (no error)"=w280) -> ("error out"=w279:errorcluster)  [unwired: 10 in]
          }
          frame "Busy" {
            n123 = call <vilib>:"Set Busy.vi"("error in (no error)"=w282) -> ("error out"=w281:errorcluster)  [unwired: 9 in, 1 out]
          }
        }
        n124 = call <vilib>:"Add State(s) to Queue__jki_lib_state_machine.vi"("State(s) in (\"\")"=w278) -> ("States Out"=w277:string)  [unwired: 14 in]
      }
      frame "UI: Front Panel State" {
        # "Argument"
        # "Set Front Panel Open or Closed\n(Usage: \"UI: Front Panel State >> Open|Close\")"
        n125 = Unbundle By Name(w285) -> ("Core.Current VI Reference"=w284:refnum<vi>)
        n126 = case shown="\"Open\", Default" w283 {
          tunnel: w287 -> [w293 w306]
          tunnel: [w295 w307] -> w286
          tunnel: w284 -> [w294 w304]
          frame "Open", Default {
            n127 = property class="VI"(reference=w294, error in=w293) -> (reference out=w291:refnum<vi>, error out=w292:errorcluster, "Front Panel.Open"=w290:bool)
            n128 = case shown="False" w290 {
              tunnel: [w298 w301] -> w295
              tunnel: w292 -> [w297 w301]
              tunnel: w291 -> [w296 _]
              frame False {
                n129 = invoke class="VI" method="FP.Open"(reference=w296, error in=w297, "Activate"=TRUE, "State"=T10."Standard") -> (error out=w298:errorcluster)  [unwired: 1 in, 4 out]
              }
              frame True {
              }
            }
          }
          frame "Close" {
            n130 = property class="VI"(reference=w304, error in=w306) -> (reference out=w303:refnum<vi>, error out=w305:errorcluster, "Front Panel.Open"=w302:bool)
            n131 = case shown="True" w302 {
              tunnel: [w308 w311] -> w307
              tunnel: w305 -> [w308 w310]
              tunnel: w303 -> [_ w309]
              frame False {
              }
              frame True {
                n132 = invoke class="VI" method="FP.Close"(reference=w309, error in=w310) -> (error out=w311:errorcluster)  [unwired: 1 in, 2 out]
              }
            }
          }
        }
        n133 = call <vilib>:"Add State(s) to Queue__jki_lib_state_machine.vi"("State(s) in (\"\")"=w289) -> ("States Out"=w288:string)  [unwired: 14 in]
      }
      frame "---------- Macro ----------" {
        # "Do not put any code in this frame.\n(It is a separator no-op. You can make a copy of this frame to create a new Macro frame)"
        n134 = call <vilib>:"Add State(s) to Queue__jki_lib_state_machine.vi"("State(s) in (\"\")"=w315) -> ("States Out"=w314:string)  [unwired: 14 in]
      }
      frame "Macro: Initialize" {
        w316 = "Data: Initialize\nInitialize Core Data\nUI: Initialize\nUI: Front Panel State >> Open"  # Data: Initialize Initialize Core Data UI: Initialize UI: Front Panel State >> Open
        # "Initialization Macro\n(This is called once, when the VI starts)"
        n135 = call <vilib>:"Add State(s) to Queue__jki_lib_state_machine.vi"("State(s) in Front (\"\")"=w316, "State(s) in (\"\")"=w320) -> ("States Out"=w319:string)  [unwired: 13 in]
      }
      frame "Macro: Exit" {
        # "Exit Macro\n(This is called once, when the VI exits)"
        n136 = Unbundle By Name(w327) -> ("Core.Close Panel on Exit?"=w326:bool)
        n137 = Select(t="UI: Front Panel State >> Close", s=w326, f="") -> (s? t:f=w323:string)
        n138 = call <vilib>:"Add State(s) to Queue__jki_lib_state_machine.vi"("State(s) in (\"\")"=w323, "State(s) at Back (\"\")"="Data: Cleanup\nExit") -> ("States Out"=w321:string)  [unwired: 13 in]
        n139 = call <vilib>:"Add State(s) to Queue__jki_lib_state_machine.vi"("State(s) in Front (\"\")"=w321, "State(s) in (\"\")"=w330) -> ("States Out"=w329:string)  [unwired: 13 in]
      }
      frame "---------- New Category ----------" {
        # "Template Separator\n(You can make a copy of, or modify, this frame)"
        n140 = call <vilib>:"Add State(s) to Queue__jki_lib_state_machine.vi"("State(s) in (\"\")"=w334) -> ("States Out"=w333:string)  [unwired: 14 in]
      }
      frame "update momenta" {
        # "Your code here.\n(You can make a copy of, or modify, this frame)"
        n141 = Greater?(x="Field::14", y=5.0) -> (0:→"Boolean":bool)
        n142 = Multiply(x="Field::14", y=9.5) -> (x*y=→"Momentum 1":dbl)
        n143 = Multiply(x="Field::14", y=3.45) -> (x*y=→"Momentum 2":dbl)
        n144 = Multiply(x="Field::14", y=3.1) -> (x*y=→"Momentum 3":dbl)
        n145 = Multiply(x="Field::14", y=2.6) -> (x*y=→"Momentum 4":dbl)
        n146 = Multiply(x="Field::14", y=2.05) -> (x*y=→"Momentum 5":dbl)
        n147 = Multiply(x="Field::14", y=1.575) -> (x*y=→"Momentum 6":dbl)
        n148 = Multiply(x="Field::14", y=1.45) -> (x*y=→"Momentum 7":dbl)
        n149 = Multiply(x="Field::14", y=1.075) -> (x*y=→"Momentum 8":dbl)
        n150 = Multiply(x="Field::14", y=0.73) -> (x*y=→"Momentum 9":dbl)
        n151 = Multiply(x="Field::14", y=0.44) -> (x*y=→"Momentum 10":dbl)
        n152 = Multiply(x="Field::14", y=0.245) -> (x*y=→"Momentum 11":dbl)
        n153 = Multiply(x="Field::14", y=0.1) -> (x*y=→"Momentum 12":dbl)
        n154 = Multiply(x="Field::14", y=0.025) -> (x*y=→"Momentum 13":dbl)
        n155 = Multiply(x="Field::14", y=0.002) -> (x*y=→"Momentum 14":dbl)
        n156 = call <vilib>:"Add State(s) to Queue__jki_lib_state_machine.vi"("State(s) in (\"\")"=w369) -> ("States Out"=w368:string)  [unwired: 14 in]
      }
      frame "tfghfh" {
        # "Your code here.\n(You can make a copy of, or modify, this frame)"
        n157 = call <vilib>:"Add State(s) to Queue__jki_lib_state_machine.vi"("State(s) in (\"\")"=w373) -> ("States Out"=w372:string)  [unwired: 14 in]
      }
      frame "y" {
        # "Your code here.\n(You can make a copy of, or modify, this frame)"
        n158 = call <vilib>:"Add State(s) to Queue__jki_lib_state_machine.vi"("State(s) in (\"\")"=w377) -> ("States Out"=w376:string)  [unwired: 14 in]
      }
      frame "jkk" {
        # "Your code here.\n(You can make a copy of, or modify, this frame)"
        n159 = call <vilib>:"Add State(s) to Queue__jki_lib_state_machine.vi"("State(s) in (\"\")"=w381) -> ("States Out"=w380:string)  [unwired: 14 in]
      }
      frame "333" {
        # "Your code here.\n(You can make a copy of, or modify, this frame)"
        n160 = call <vilib>:"Add State(s) to Queue__jki_lib_state_machine.vi"("State(s) in (\"\")"=w385) -> ("States Out"=w384:string)  [unwired: 14 in]
      }
      frame "555" {
        # "Your code here.\n(You can make a copy of, or modify, this frame)"
        n161 = call <vilib>:"Add State(s) to Queue__jki_lib_state_machine.vi"("State(s) in (\"\")"=w389) -> ("States Out"=w388:string)  [unwired: 14 in]
      }
    }
  }
